vi "Format Metric.vi"(10 "Metric name":string, 11 "Metric properties":T1) -> (3 "Metrics string":string)   [LabVIEW 2015, in "NI_Azure_Blob.lvlib"]
uses:
  NI_Azure_Blob.lvlib
  Metrics.ctl
  Retention Policy.ctl
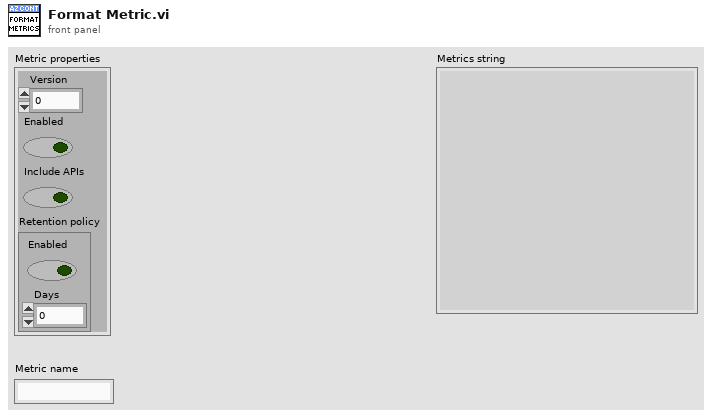
[diagram p1: front panel]
types:
  T1 = typedef "NI_Azure_Blob.lvlib/Metrics.ctl" = cluster{"Version":dbl, "Enabled":bool, "Include APIs":bool, "Retention policy":T2}
  T2 = typedef "NI_Azure_Blob.lvlib/Retention Policy.ctl" = cluster{"Enabled":bool, "Days":u32}
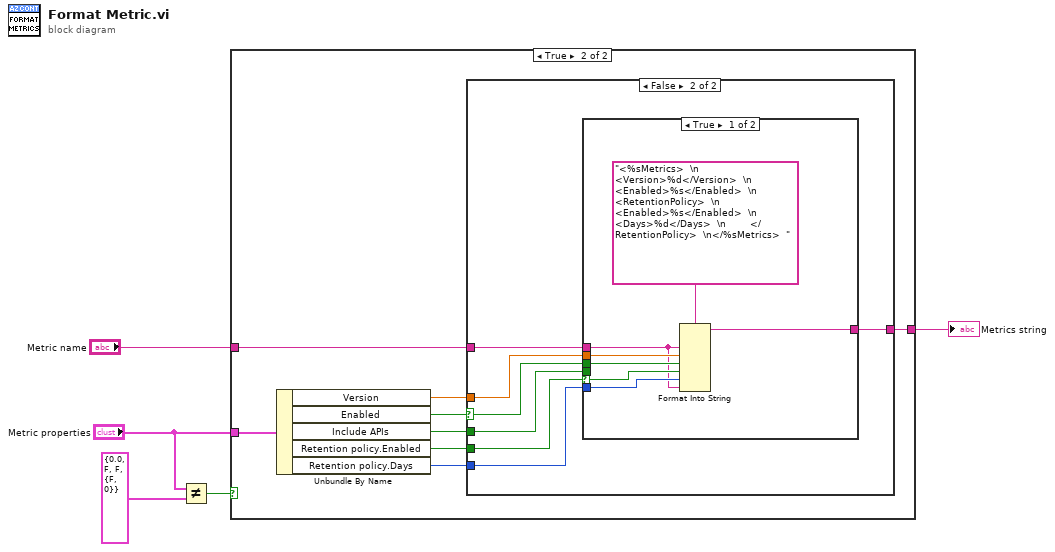
[diagram p0: block diagram]
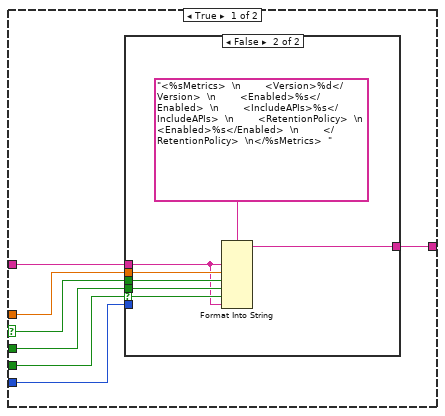
[diagram p3: hidden frame]
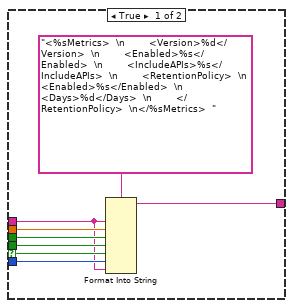
[diagram p4: hidden frame]
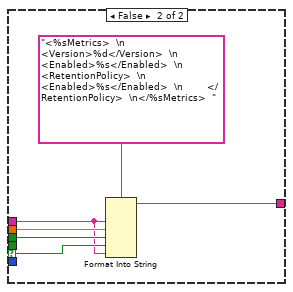
[diagram p5: hidden frame]
diagram:
  n1 = Not Equal?(x="Metric properties", y=T1 {"Version"=0.0, "Enabled"=FALSE, "Include APIs"=FALSE, "Retention policy"={"Enabled"=FALSE, "Days"=0}}) -> (x != y?=w5:bool)
  n2 = case shown="True" w5 {
    tunnel: "Metric properties" -> [_ w13]
    tunnel: [_ w12] -> w3
    tunnel: "Metric name" -> [_ w6]
    frame False {
    }
    frame True {
      n3 = Unbundle By Name(w13) -> ("Version"=w11:dbl, "Enabled"=w10:bool, "Include APIs"=w9:bool, "Retention policy.Enabled"=w8:bool, "Retention policy.Days"=w7:u32)
      n4 = case shown="False" w10 {
        selector: w10 -> [w18 w40]
        tunnel: [w20 w42] -> w12
        tunnel: w11 -> [w19 w41]
        tunnel: w8 -> [w16 w38]
        tunnel: w7 -> [w15 w37]
        tunnel: w6 -> [w14 w36]
        tunnel: w9 -> [w17 w39]
        frame True {
          n5 = case shown="False" w16 {
            selector: w16 -> [w23 w30]
            tunnel: [w27 w34] -> w20
            tunnel: w19 -> [w26 w33]
            tunnel: w18 -> [w25 w32]
            tunnel: w17 -> [w24 w31]
            tunnel: w15 -> [w22 _]
            tunnel: w14 -> [w21 w29]
            frame True {
              n6 = Format Into String(format string="<%sMetrics>  \n        <Version>%d</Version>  \n        <Enabled>%s</Enabled>  \n        <IncludeAPIs>%s</IncludeAPIs>  \n        <RetentionPolicy>  \n            <Enabled>%s</Enabled>  \n            <Days>%d</Days>  \n        </RetentionPolicy>  \n</%sMetrics>  ", w21, w26, w25, w24, w23, w22, w21) -> (resulting string=w27:string)  [unwired: 2 in, 1 out]
            }
            frame False {
              n7 = Format Into String(format string="<%sMetrics>  \n        <Version>%d</Version>  \n        <Enabled>%s</Enabled>  \n        <IncludeAPIs>%s</IncludeAPIs>  \n        <RetentionPolicy>  \n            <Enabled>%s</Enabled>  \n        </RetentionPolicy>  \n</%sMetrics>  ", w29, w33, w32, w31, w30, w29) -> (resulting string=w34:string)  [unwired: 2 in, 1 out]
            }
          }
        }
        frame False {
          n8 = case shown="True" w38 {
            selector: w38 -> [w45 w51]
            tunnel: [w48 w54] -> w42
            tunnel: w41 -> [w47 w53]
            tunnel: w40 -> [w46 w52]
            tunnel: w39 -> [_ _]
            tunnel: w37 -> [w44 _]
            tunnel: w36 -> [w43 w50]
            frame True {
              n9 = Format Into String(format string="<%sMetrics>  \n        <Version>%d</Version>  \n        <Enabled>%s</Enabled>  \n        <RetentionPolicy>  \n            <Enabled>%s</Enabled>  \n            <Days>%d</Days>  \n        </RetentionPolicy>  \n</%sMetrics>  ", w43, w47, w46, w45, w44, w43) -> (resulting string=w48:string)  [unwired: 2 in, 1 out]
            }
            frame False {
              n10 = Format Into String(format string="<%sMetrics>  \n        <Version>%d</Version>  \n        <Enabled>%s</Enabled>  \n        <RetentionPolicy>  \n            <Enabled>%s</Enabled>  \n        </RetentionPolicy>  \n</%sMetrics>  ", w50, w53, w52, w51, w50) -> (resulting string=w54:string)  [unwired: 2 in, 1 out]
            }
          }
        }
      }
    }
  }
  "Metrics string" <- w3
